vi "test_phase_calibration.vi"() -> ()   [LabVIEW 2009]
doc: "Copyright (c) 2010 Stepan A. Baranov (stepan@baranov.su)\nAll rights reserved.\nweb-site: www.OCTLab.org"
uses:
  OCTLib_64.dll
panel:
  out "error out":errorcluster
  out "level":i32
  out "width":i32
  out "height":i32
  in  "Small/Big":bool
  out "loop #":i32
  out "RSM_STAT time":u32
  out "LabView time":u32
  out "RSM_STAT Array":dbl[][](array[numeric])
  out "LabView Array":dbl[][](array[numeric])
  in  "stop":bool
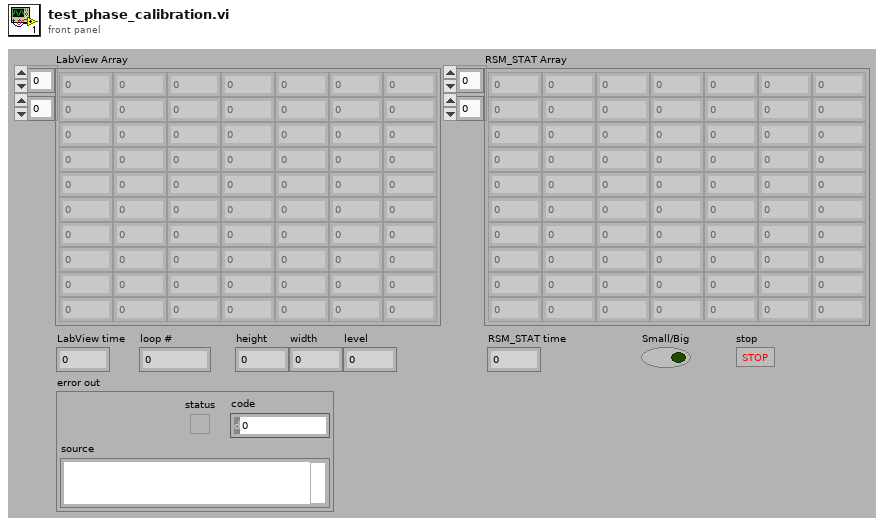
[diagram p1: front panel]
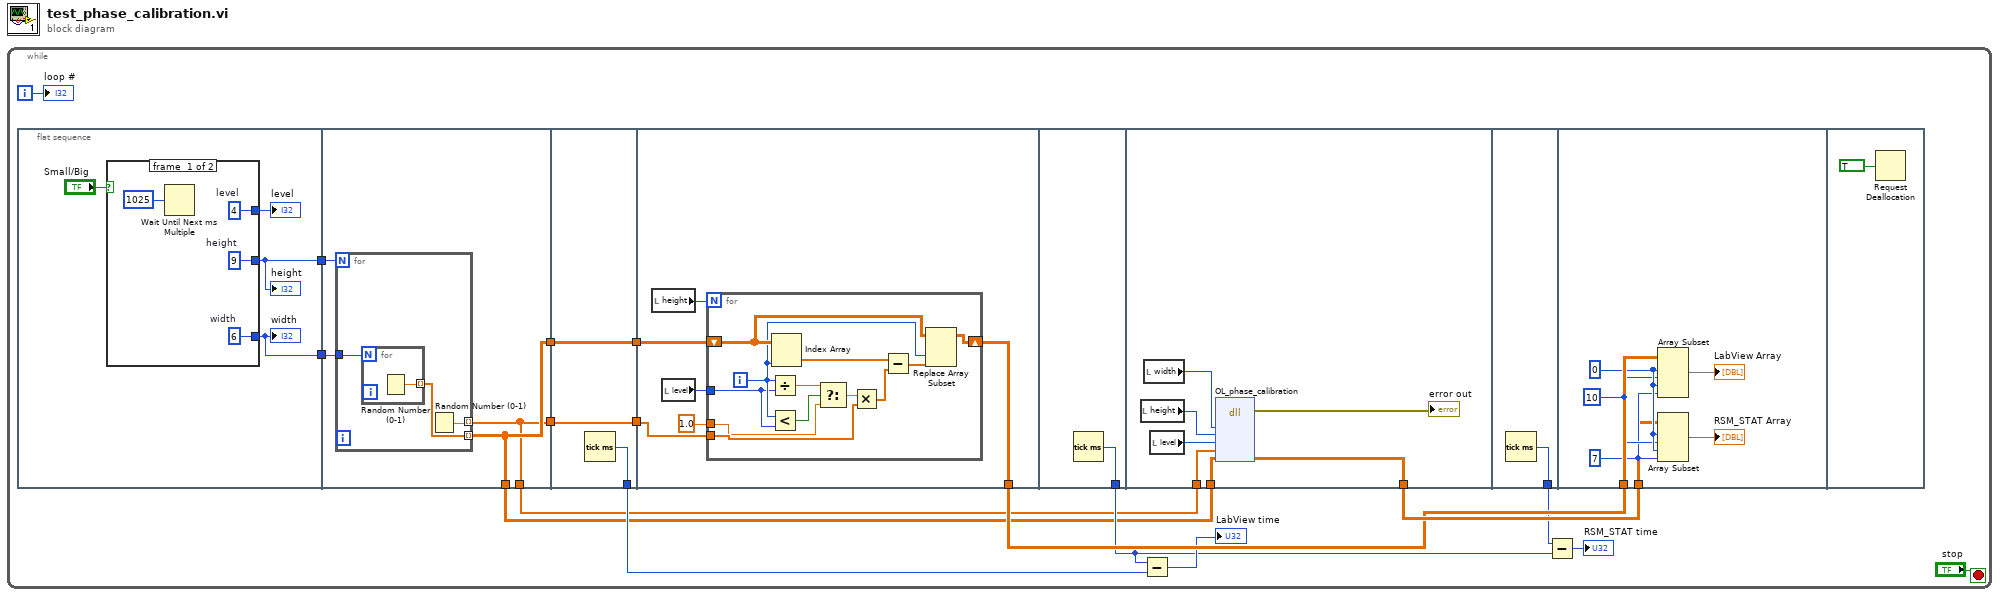
[diagram p0: block diagram]
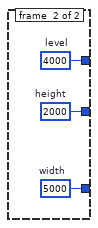
[diagram p2: hidden frame]
diagram:
  n1 = while {
    i -> [w9]
    stop <- "stop" stop-if-true
    n2 = flat-sequence {
      tunnel: [w20] -> w2
      tunnel: [w19] -> w1
      tunnel: [w30] -> w8
      tunnel: [w29] -> w7
      tunnel: [w30] -> w5
      tunnel: [w29] -> w3
      tunnel: w2 -> [w32]
      tunnel: w1 -> [w31]
      tunnel: [w39] -> w14
      tunnel: [w38] -> w6
      tunnel: w5 -> [w38]
      tunnel: [w37] -> w4
      tunnel: w3 -> [w37]
      tunnel: [w45] -> w15
      tunnel: w6 -> [w44]
      tunnel: w4 -> [w43]
      tunnel: [w58] -> w11
      tunnel: w8 -> [w65]
      tunnel: [w64] -> w16
      tunnel: w7 -> [w63]
      tunnel: [w66] -> w12
      tunnel: w16 -> [w67]
      tunnel: w15 -> [w73]
      frame #0 {
        n3 = case shown="False" "Small/Big" {
          tunnel: [w23 w28] -> w19
          tunnel: [w24 w27] -> w20
          tunnel: [w25 w26] -> w18
          frame #0 {
            w25 = 4  # level
            w24 = 6  # width
            w23 = 9  # height
            n4 = Wait Until Next ms Multiple(millisecond multiple=u32 1025) -> ()  [unwired: 1 out]
          }
          frame #1 {
            w26 = 4000  # level
            w27 = 5000  # width
            w28 = 2000  # height
          }
        }
        "height" <- w19
        "width" <- w20
        "level" <- w18
      }
      frame #1 {
        n5 = for {
          N: w31 -> [_]
          tunnel: w32 -> [w35]
          tunnel: [w34] -> w30 mode=indexing
          tunnel: [w33] -> w29 mode=indexing
          n6 = for {
            N: w35 -> [_]
            tunnel: [w36] -> w34 mode=indexing
            n7 = Random Number (0-1)() -> (number: 0 to 1=w36:dbl)
          }
          n8 = Random Number (0-1)() -> (number: 0 to 1=w33:dbl)
        }
      }
      frame #2 {
        n9 = Tick Count (ms)() -> (millisecond timer value=w39:u32)
      }
      frame #3 {
        n10 = local read "height"() -> (w42:i32)
        n11 = local read "level"() -> (w41:i32)
        n12 = for {
          N: w42 -> [_]
          tunnel: w43 -> [w54]
          shift-right: [w49] -> w45
          shift-left: w44 -> [w51]
          tunnel: w41 -> [w47]
          tunnel: 1.0 ("f") -> [w46]
          i -> [w48]
          n13 = Divide(x=w48, y=w47) -> (x/y=w56:dbl)
          n14 = Less?(x=w48, y=w47) -> (x < y?=w57:bool)
          n15 = Index Array(array=w51, index (col)=w48) -> (element=w53:dbl[])  [unwired: 1 in]
          n16 = Select(t=w56, s=w57, f=w46) -> (s? t:f=w55:dbl)
          n17 = Multiply(x=w55, y=w54) -> (x*y=w52:dbl[])
          n18 = Subtract(x=w53, y=w52) -> (x-y=w50:dbl[])
          n19 = Replace Array Subset(array=w51, new element=w50, index (col)=w48) -> (w49:dbl[][])  [unwired: 1 in]
        }
      }
      frame #4 {
        n20 = Tick Count (ms)() -> (millisecond timer value=w58:u32)
      }
      frame #5 {
        n21 = local read "height"() -> (w61:i32)
        n22 = local read "width"() -> (w62:i32)
        n23 = local read "level"() -> (w60:i32)
        n24 = dll-call lib="OCTLib**.*" fn="OL_phase_calibration"("width"=w62, "height"=w61, "level"=w60, "ref"=w63, "data"=w65) -> (error out=→"error out":errorcluster, "data"=w64:dbl[][])  [unwired: 8 in, 1 out]
      }
      frame #6 {
        n25 = Tick Count (ms)() -> (millisecond timer value=w66:u32)
      }
      frame #7 {
        w70 = 10 ("length")
        w69 = 7 ("length")
        w71 = 0 ("index")
        n26 = Array Subset(array=w73, index (row)=w71, length (row)=w70, index (col)=w71, length (col)=w69) -> (→"LabView Array":dbl[][])
        n27 = Array Subset(array=w67, index (row)=w71, length (row)=w70, index (col)=w71, length (col)=w69) -> (→"RSM_STAT Array":dbl[][])
      }
      frame #8 {
        n28 = Request Deallocation(TRUE ("flag")) -> ()
      }
    }
    n29 = Subtract(x=w11, y=w14) -> (x-y=→"LabView time":u32)
    n30 = Subtract(x=w12, y=w11) -> (x-y=→"RSM_STAT time":u32)
    "loop #" <- w9
  }
